vi "cdaq_anal_open.vi"(8 "error in":errorcluster, 11 "cdaq session in":T1={"mclk [Hz]"=12800000.0, "DAC device"="", "ADC device"="", "DAC task"="", "ADC task"="", "adc idn"="", "dac idn"="", "fs [Hz]"=50000.0, "queue adc cmd"=refnum, "queue adc data"=refnum, "adc proc ref"=refnum}) -> (0 "error out":errorcluster, 1 "DAC idn":string, 2 "ADC idn":string, 3 "cdaq session out":T1={"mclk [Hz]"=12800000.0, "DAC device"="", "ADC device"="", "DAC task"="", "ADC task"="", "adc idn"="", "dac idn"="", "fs [Hz]"=50000.0, "queue adc cmd"=refnum, "queue adc data"=refnum, "adc proc ref"=refnum})   [LabVIEW 2020]
uses:
  cdaq_anal_session.ctl
  cdaq_anal_adc_command.ctl
  cdaq_anal_adc_data.ctl
  <vilib>/Utility/error.llb/Error Cluster From Error Code.vi
  <vilib>/DAQmx/create/channels.llb/DAQmx Create Channel (AI-Voltage-Basic).vi
  <vilib>/DAQmx/configure/timing.llb/DAQmx Timing (Sample Clock).vi
  <vilib>/DAQmx/create/channels.llb/DAQmx Create Channel (AO-Voltage-Basic).vi
  <vilib>/ErrorRing/Error Ring.xnode
  <resource>/objmgr/daqmx.rc
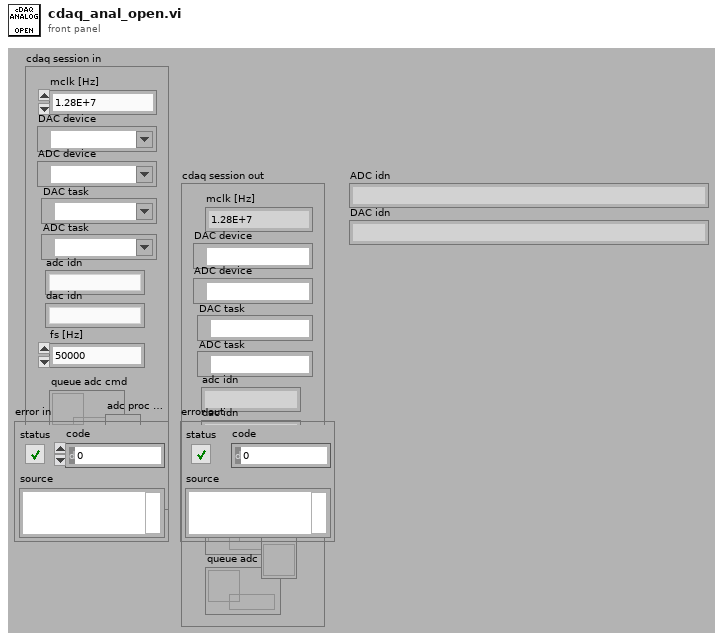
[diagram p1: front panel]
types:
  T1 = typedef "cdaq_anal_session.ctl" = cluster{"mclk [Hz]":dbl, "DAC device":tag, "ADC device":tag, "DAC task":refnum<k21>, "ADC task":refnum<k21>, "adc idn":string, "dac idn":string, "fs [Hz]":dbl, "queue adc cmd":refnum<queue>, "queue adc data":refnum<queue>, "adc proc ref":refnum<vi>}
  T2 = typedef "cdaq_anal_adc_data.ctl" = cluster{"wave":dbl[][], "timestamp [s]":dbl, "abs timestamp":timestamp, "Aborted":bool}
  T3 = typedef "cdaq_anal_adc_command.ctl" = cluster{"sample to get":i32, "stop":bool, "abort":bool}
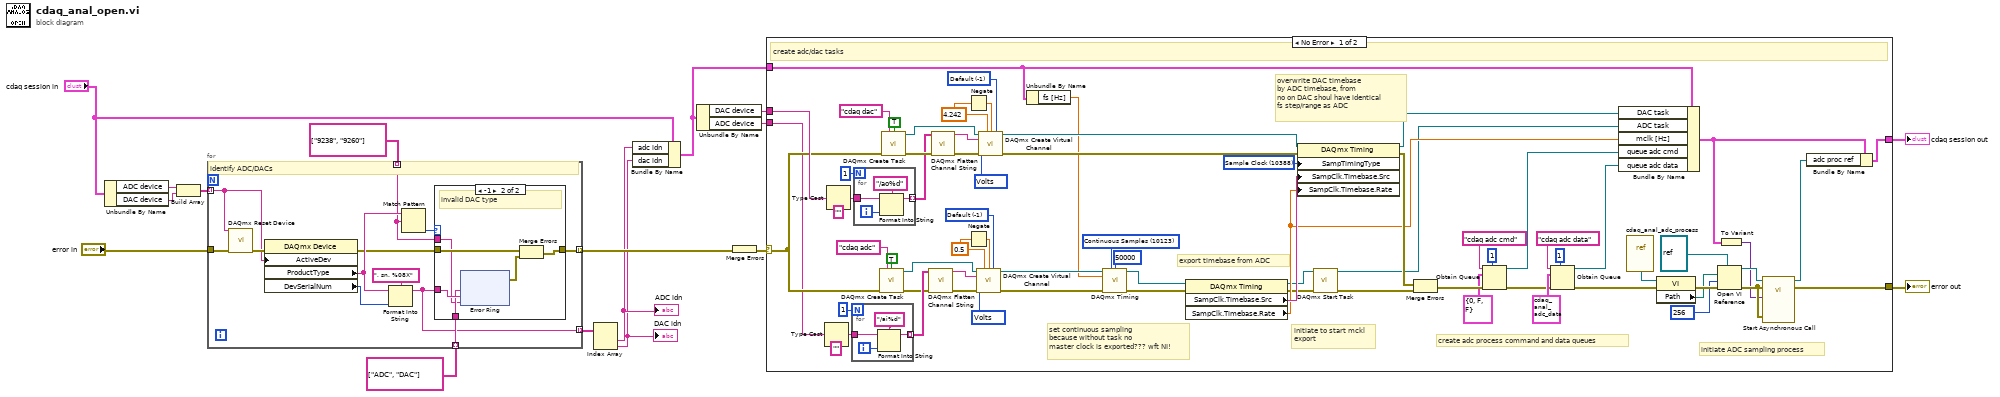
[diagram p0: block diagram]
diagram:
  n1 = Unbundle By Name("cdaq session in") -> ("ADC device"=w16:tag, "DAC device"=w15:tag)
  n2 = Build Array(w16, w15) -> (w14:tag[])
  n3 = for {
    tunnel: w14 -> [w28] mode=indexing
    tunnel: "error in" -> [w22]
    tunnel: string[] ["ADC", "DAC"] -> [w21] mode=indexing
    tunnel: string[] ["9238", "9260"] -> [w18] mode=indexing
    tunnel: [w20] -> w11 mode=indexing
    tunnel: [w19] -> w3 mode=indexing
    # "identify ADC/DACs"
    n4 = call <vilib>:"DAQmx Reset Device.vi"("device in"=w28, "error in"=w22) -> ("error out"=w29:errorcluster)  [unwired: 13 in]
    n5 = property class="DAQmx Device"(error in=w29, "ActiveDev"=w28) -> (error out=w23:errorcluster, "ProductType"=w25:string, "DevSerialNum"=w27:u32)  [unwired: 1 in, 1 out]
    n6 = Format Into String(format string=", sn. %08X", initial string=w25, w27) -> (resulting string=w19:string)  [unwired: 1 in, 1 out]
    n7 = Match Pattern(string=w25, regular expression=w18) -> (offset past match=w24:i32)  [unwired: 1 in, 3 out]
    n8 = case shown="-1" w24 {
      tunnel: w23 -> [w30 w36]
      tunnel: w19 -> [_ w33]
      tunnel: [w30 w34] -> w20
      tunnel: w21 -> [_ w32]
      tunnel: w18 -> [_ w31]
      frame Default {
      }
      frame -1 {
        # "invalid DAC type"
        n9 = xnode "Error Ring"("parameter 0"=w32, "parameter 1"=w33, "parameter 2"=w31) -> ("error out"=w35:errorcluster)
        n10 = Merge Errors(w36, w35) -> (w34:errorcluster)
      }
    }
  }
  n11 = Index Array(array=w3) -> (element #1=w2:string, element #2=w1:string)  [unwired: 2 in]
  "ADC idn" <- w2
  "DAC idn" <- w1
  n12 = Bundle By Name(cluster="cdaq session in", "adc idn"=w2, "dac idn"=w1) -> (w4:T1)
  n13 = Unbundle By Name(w4) -> ("DAC device"=w9:tag, "ADC device"=w8:tag)
  n14 = Merge Errors(w11) -> (w10:errorcluster)
  n15 = case shown="No Error" w10 {
    selector: w10 -> [w93 w127]
    tunnel: w9 -> [w108 _]
    tunnel: w4 -> [w74 w128]
    tunnel: w8 -> [w92 _]
    tunnel: [w49 w127] -> w7
    tunnel: [w46 w128] -> w6
    frame No Error {
      w75 = 10388 items=["Sample Clock"=10388, "Burst Handshake"=12548, "Handshake"=10389, "Implicit"=10451, "On Demand"=10390, "Change Detection"=12504, "Pipelined Sample Clock"=14668] ("SampTimingType")
      w83 = 10123 items=["Finite Samples"=10178, "Continuous Samples"=10123, "Hardware Timed Single Point"=12522] ("sample mode")
      w88 = 4.242 ("maximum value")
      w91 = 0.5 ("maximum value")
      w105 = -1 items=["Default"=-1, "RSE"=10083, "Differential"=10106, "Pseudodifferential"=12529] ("output terminal configuration")
      w100 = 10348 items=["Volts"=10348, "From Custom Scale"=10065] ("units")
      w106 = -1 items=["Default"=-1, "RSE"=10083, "Differential"=10106, "Pseudodifferential"=12529] ("output terminal configuration")
      w112 = 10348 items=["Volts"=10348, "From Custom Scale"=10065] ("units")
      # "initiate ADC sampling process"
      # "create adc process command and data queues"
      # "initiate to start mckl\nexport"
      # "set continuous sampling\nbecause without task no\nmaster clock is exported??? wft NI!"
      # "overwrite DAC timebase\nby ADC timebase, from\nno on DAC shoul have identical\nfs step/range as ADC"
      # "export timebase from ADC"
      # "create adc/dac tasks"
      n16 = Type Cast(type="", x=w92) -> (*(type *) &x=w102:string)
      n17 = Type Cast(type="", x=w108) -> (*(type *) &x=w110:string)
      n18 = for {
        N: 1 -> [_]
        tunnel: w102 -> [w121]
        tunnel: [w119] -> w98 mode=indexing
        i -> [w120]
        n19 = Format Into String(format string="/ai%d", initial string=w121, w120) -> (resulting string=w119:string)  [unwired: 1 in, 1 out]
      }
      n20 = for {
        N: 1 -> [_]
        tunnel: w110 -> [w125]
        tunnel: [w123] -> w114 mode=indexing
        i -> [w124]
        n21 = Format Into String(format string="/ao%d", initial string=w125, w124) -> (resulting string=w123:string)  [unwired: 1 in, 1 out]
      }
      n22 = call <vilib>:"DAQmx Create Task.vi"("new task name"="cdaq adc", "auto cleanup"=TRUE, "error in"=w93) -> ("task out"=w95:refnum<k21>, "error out"=w96:errorcluster)  [unwired: 11 in]
      n23 = call <vilib>:"DAQmx Create Task.vi"("new task name"="cdaq dac", "auto cleanup"=TRUE, "error in"=w93) -> ("task out"=w117:refnum<k21>, "error out"=w116:errorcluster)  [unwired: 11 in]
      n24 = call <vilib>:"DAQmx Flatten Channel String.vi"("names in"=w98, "error in"=w96) -> ("names out"=w99:string, "error out"=w97:errorcluster)  [unwired: 12 in]
      n25 = call <vilib>:"DAQmx Flatten Channel String.vi"("names in"=w114, "error in"=w116) -> ("names out"=w113:string, "error out"=w115:errorcluster)  [unwired: 12 in]
      n26 = Negate(x=w88) -> (-x=w89:dbl)
      n27 = Negate(x=w91) -> (-x=w90:dbl)
      n28 = call-poly <vilib>:"DAQmx Create Virtual Channel.vi"("task in"=w95, "maximum value"=w91, "minimum value"=w90, "input terminal configuration"=w105, "physical channels"=w99, "units"=w100, "error in"=w97) -> ("task out"=w80:refnum<k21>, "error out"=w81:errorcluster)  [unwired: 7 in]
      n29 = call-poly <vilib>:"DAQmx Create Virtual Channel.vi"("task in"=w117, "maximum value"=w88, "minimum value"=w89, "output terminal configuration"=w106, "physical channels"=w113, "units"=w112, "error in"=w115) -> ("task out"=w76:refnum<k21>, "error out"=w77:errorcluster)  [unwired: 7 in]
      n30 = Unbundle By Name(w74) -> ("fs [Hz]"=w73:dbl)
      n31 = call-poly <vilib>:"DAQmx Timing.vi"("task/channels in"=w80, "sample mode"=w83, "samples per channel"=50000, "rate"=w73, "error in"=w81) -> ("task out"=w78:refnum<k21>, "error out"=w79:errorcluster)  [unwired: 9 in]
      n32 = property class="DAQmx Timing"(reference=w78, error in=w79) -> (reference out=w71:refnum<k21>, error out=w72:errorcluster, "SampClk.Timebase.Src"=w87:tag, "SampClk.Timebase.Rate"=w84:dbl)
      n33 = property class="DAQmx Timing"(reference=w76, error in=w77, "SampTimingType"=w75, "SampClk.Timebase.Src"=w87, "SampClk.Timebase.Rate"=w84) -> (reference out=w85:refnum<k21>, error out=w86:errorcluster)
      n34 = call <vilib>:"DAQmx Start Task.vi"("task/channels in"=w71, "error in"=w72) -> ("task out"=w59:refnum<k21>, "error out"=w70:errorcluster)  [unwired: 12 in]
      n35 = Merge Errors(w86, w70) -> (w69:errorcluster)
      n36 = Obtain Queue(max queue size (-1, unlimited)=1, name (unnamed)="cdaq adc cmd", element data type=T3 {"sample to get"=0, "stop"=FALSE, "abort"=FALSE} ("adc cmd"), error in (no error)=w69) -> (queue out=w61:refnum<queue>, error out=w62:errorcluster)  [unwired: 1 in, 1 out]
      n37 = Obtain Queue(max queue size (-1, unlimited)=1, name (unnamed)="cdaq adc data", element data type=T2 {"wave"=[], "timestamp [s]"=0.0, "abs timestamp"=timestamp(0 s since 1904-01-01), "Aborted"=FALSE} ("adc data"), error in (no error)=w62) -> (queue out=w60:refnum<queue>, error out=w50:errorcluster)  [unwired: 1 in, 1 out]
      n38 = Bundle By Name(cluster=w74, "DAC task"=w85, "ADC task"=w59, "mclk [Hz]"=w84, "queue adc cmd"=w61, "queue adc data"=w60) -> (w48:T1)
      n39 = vi-ref "cdaq_anal_adc_process.vi"() -> (w57:refnum<vi>)
      n40 = property class="VI"(reference=w57, error in=w50) -> (error out=w56:errorcluster, "Path"=w54:path)  [unwired: 1 out]
      n41 = Open VI Reference(type specifier VI Refnum (for type only)=refnum<vi> refnum, vi path=w54, options=256, error in (no error)=w56) -> (vi reference=w58:refnum<vi>, error out=w55:errorcluster)  [unwired: 2 in]
      n42 = To Variant(anything=w48) -> (Variant=w51:variant)
      n43 = call-by-ref "Start Asynchronous Call"(reference=w58, error in=w55, "error in"=w55, "cdaq session"=w51) -> (reference out=w47:refnum<vi>, error out=w49:errorcluster)  [unwired: 9 in, 1 out]
      n44 = Bundle By Name(cluster=w48, "adc proc ref"=w47) -> (w46:T1)
    }
    frame Error {
    }
  }
  "cdaq session out" <- w6
  "error out" <- w7
